vi "(SubVI) Faxen's law_YCC.vi"(3 "viscosity (cP)":dbl=1.0, 4 "bead height (um)":dbl=1.0, 5 "bead radius (um)":dbl=0.515) -> (1 "Faxen's law of friction coefficient (N/(m/s))":dbl)   [LabVIEW 2014]
panel:
  out "Drag Coefficient N/(m/s)":dbl
  out "Faxen's correction N/(m/s)":dbl
  out "x*y":dbl
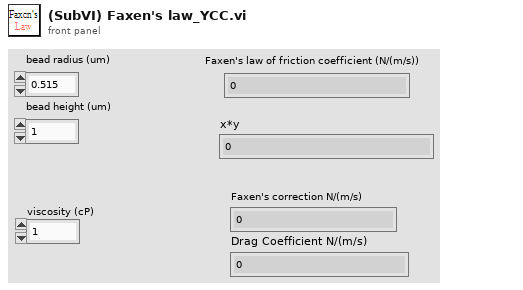
[diagram p1: front panel]
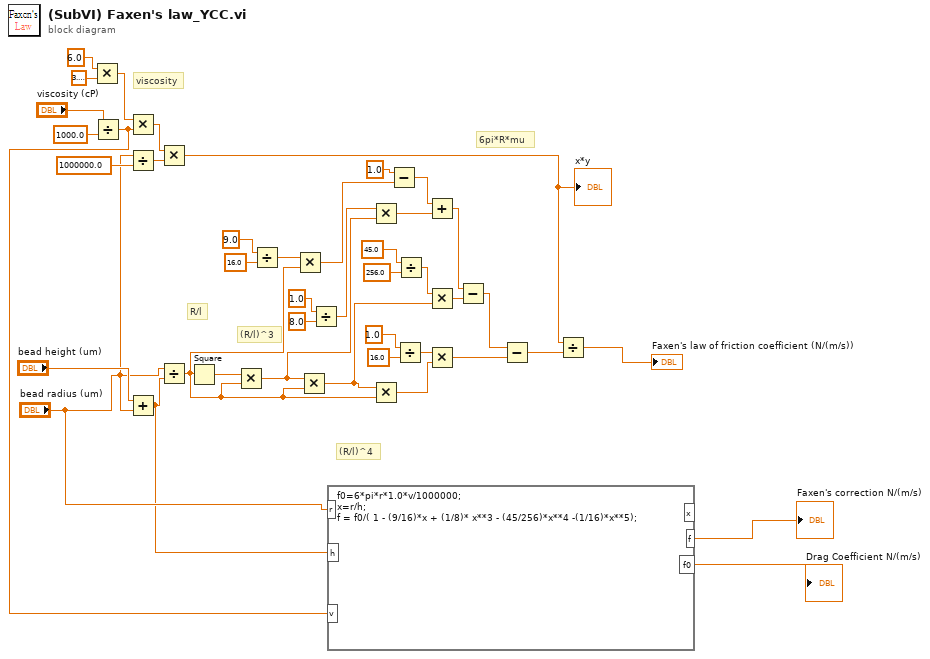
[diagram p0: block diagram]
diagram:
  # "viscosity"
  # "6pi*R*mu"
  # "(R/l)^4"
  # "(R/l)^3"
  # "R/l"
  n1 = Multiply(x=6.0, y=3.141592653589793) -> (x*y=w39:dbl)
  n2 = Divide(x="viscosity (cP)", y=1000.0) -> (x/y=w5:dbl)
  n3 = Multiply(x=w39, y=w5) -> (x*y=w38:dbl)
  n4 = Divide(x="bead radius (um)", y=1000000.0) -> (x/y=w10:dbl)
  n5 = Add(x="bead height (um)", y="bead radius (um)") -> (x+y=w1:dbl)
  n6 = Multiply(x=w38, y=w10) -> (x*y=w9:dbl)
  "x*y" <- w9
  n7 = Divide(x="bead radius (um)", y=w1) -> (x/y=w17:dbl)
  n8 = Square(x=w17) -> (x^2=w26:dbl)
  n9 = Multiply(x=w26, y=w17) -> (x*y=w22:dbl)
  n10 = Divide(x=9.0, y=16.0) -> (x/y=w29:dbl)
  n11 = Multiply(x=w29, y=w17) -> (x*y=w27:dbl)
  n12 = Multiply(x=w22, y=w17) -> (x*y=w18:dbl)
  n13 = Divide(x=1.0, y=8.0) -> (x/y=w25:dbl)
  n14 = formula code="f0=6*pi*r*1.0*v/1000000;\nx=r/h;\nf = f0/( 1 - (9/16)*x + (1/8)* x**3 - (45/256)*x**4 -(1/16)*x**5);"("r"="bead radius (um)", "h"=w1, "v"=w5) -> ("f"=→"Faxen's correction N/(m/s)":dbl, "f0"=→"Drag Coefficient N/(m/s)":dbl)  [unwired: 1 out]
  n15 = Multiply(x=w25, y=w22) -> (x*y=w23:dbl)
  n16 = Multiply(x=w18, y=w17) -> (x*y=w15:dbl)
  n17 = Subtract(x=1.0, y=w27) -> (x-y=w24:dbl)
  n18 = Divide(x=1.0, y=16.0) -> (x/y=w16:dbl)
  n19 = Divide(x=45.0, y=256.0) -> (x/y=w21:dbl)
  n20 = Add(x=w24, y=w23) -> (x+y=w19:dbl)
  n21 = Multiply(x=w21, y=w18) -> (x*y=w20:dbl)
  n22 = Multiply(x=w16, y=w15) -> (x*y=w13:dbl)
  n23 = Subtract(x=w19, y=w20) -> (x-y=w14:dbl)
  n24 = Subtract(x=w14, y=w13) -> (x-y=w12:dbl)
  n25 = Divide(x=w9, y=w12) -> (x/y=→"Faxen's law of friction coefficient (N/(m/s))":dbl)
